vi "Linecut.vi"(5 "linecut y position":dbl, 7 "linecut x position":dbl, 8 "error in (no error)":errorcluster, 9 "Linear/Log":u16(ring) items=["Linear", "Log"], 10 "Linecut direction (fast/slow)":u8(ring) items=["fast", "slow"], 11 "Input image":dbl[][](graph)) -> (0 "error out":errorcluster, 3 "Linecut profile":dbl[](graph))   [LabVIEW 2014]
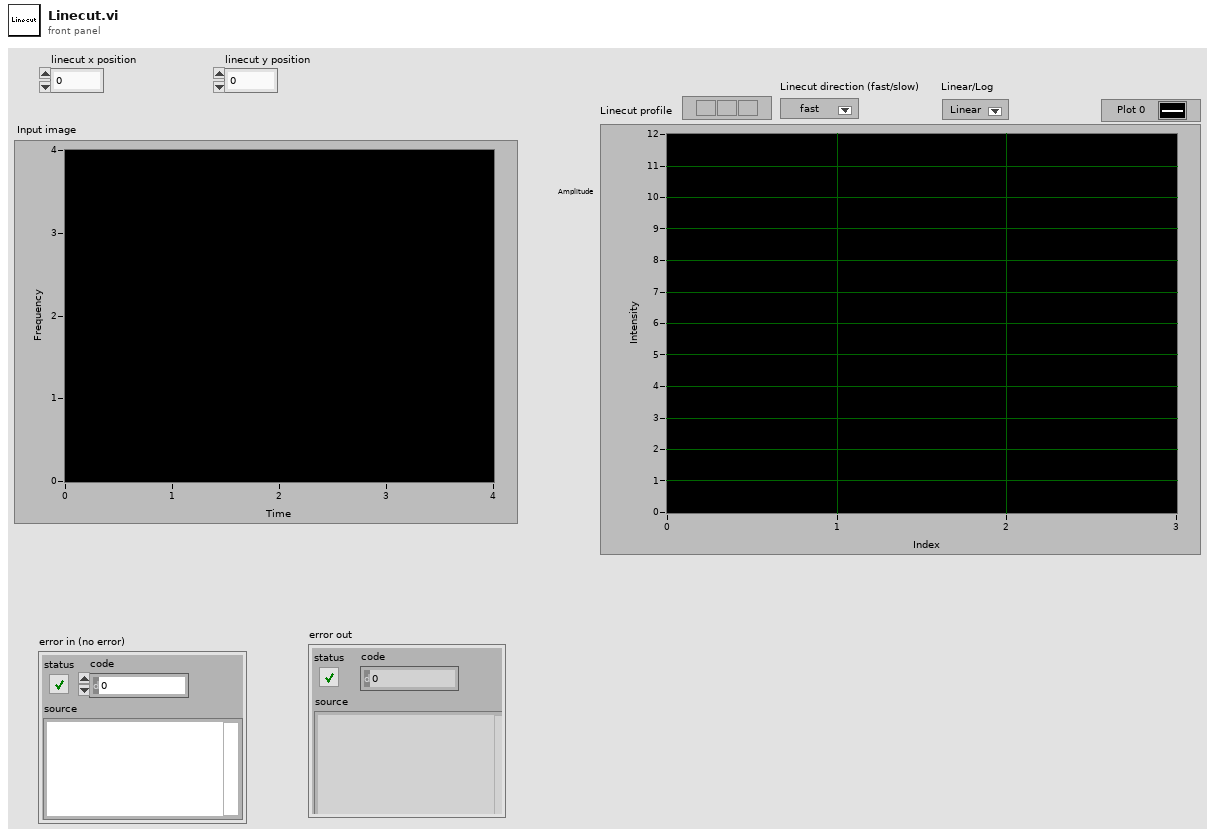
[diagram p1: front panel]
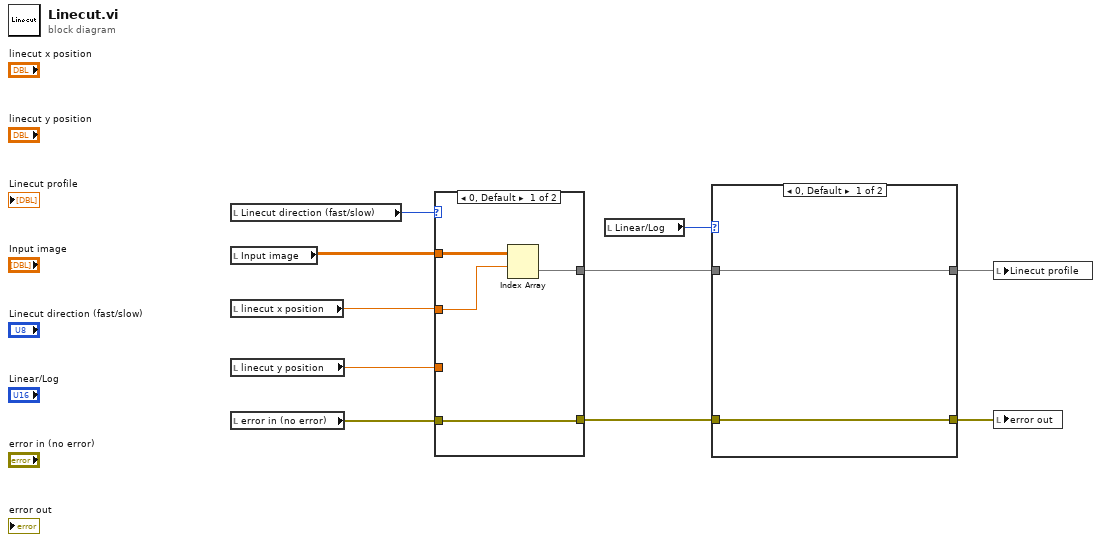
[diagram p0: block diagram]
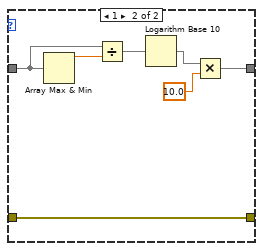
[diagram p2: hidden frame]
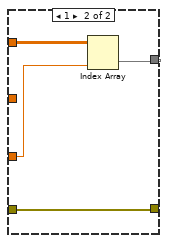
[diagram p3: hidden frame]
diagram:
  n1 = local read "Linecut direction (fast/slow)"() -> (w8:u8)
  n2 = local read "Input image"() -> (w7:dbl[][])
  n3 = local read "linecut x position"() -> (w2:dbl)
  n4 = local read "linecut y position"() -> (w1:dbl)
  n5 = local read "error in (no error)"() -> (w4:errorcluster)
  n6 = case shown="0, Default" w8 {
    tunnel: w7 -> [w14 w18]
    tunnel: w2 -> [w13 _]
    tunnel: w1 -> [_ w17]
    tunnel: [w12 w16] -> w10
    tunnel: [w11 w15] -> w9
    tunnel: w4 -> [w11 w15]
    frame 0, Default {
      n7 = Index Array(array=w14, index (row)=w13) -> (element=w12:dbl[])  [unwired: 1 in]
    }
    frame 1 {
      n8 = Index Array(array=w18, index (col)=w17) -> (element=w16:dbl[])  [unwired: 1 in]
    }
  }
  n9 = local read "Linear/Log"() -> (w6:u16)
  n10 = case shown="0, Default" w6 {
    tunnel: w10 -> [w20 w26]
    tunnel: [w20 w22] -> w5
    tunnel: w9 -> [w19 w21]
    tunnel: [w19 w21] -> w3
    frame 0, Default {
    }
    frame 1 {
      n11 = Array Max & Min(array=w26) -> (max value=w27:dbl)  [unwired: 3 out]
      n12 = Divide(x=w26, y=w27) -> (x/y=w25:dbl[])
      n13 = Logarithm Base 10(1:w25) -> (0:w24:dbl[])
      n14 = Multiply(x=w24, y=10.0) -> (x*y=w22:dbl[])
    }
  }
  n15 = local write "Linecut profile"(w5) -> ()
  n16 = local write "error out"(w3) -> ()
